vi "Pi divided by 4.vi"() -> (0 "Pi/4":dbl=4.0 format="%#_13g")   [LabVIEW 2016]
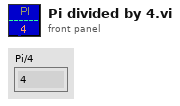
[diagram p1: front panel]
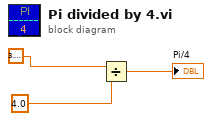
[diagram p0: block diagram]
diagram:
  n1 = Divide(x=3.141592653589793, y=4.0) -> (x/y=→"Pi/4":dbl)
